vi "Test_User_Event.vi"() -> ()   [LabVIEW 2014, in "User_Event_Library.lvlib"]
uses:
  User_Event_Library.lvlib
  Send_User_Event_Array.vi
panel:
  out "number (0 to 1)":dbl(graph)
  in  "Blank Button":bool
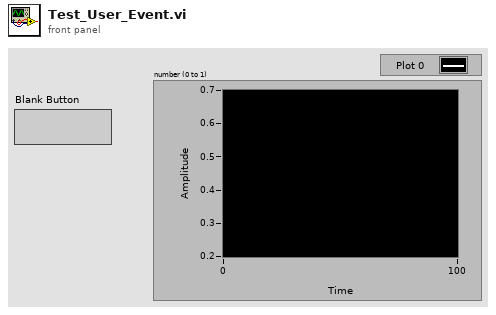
[diagram p1: front panel]
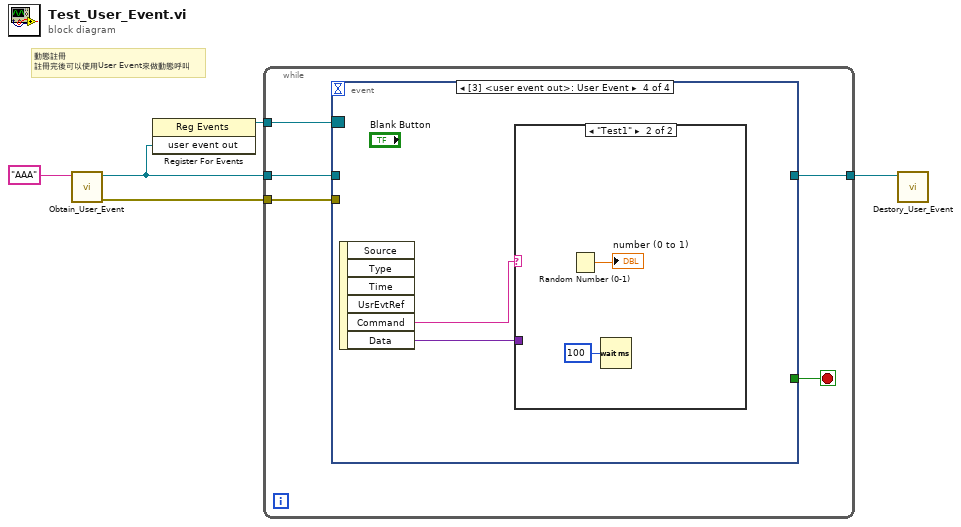
[diagram p0: block diagram]
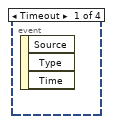
[diagram p2: hidden frame]
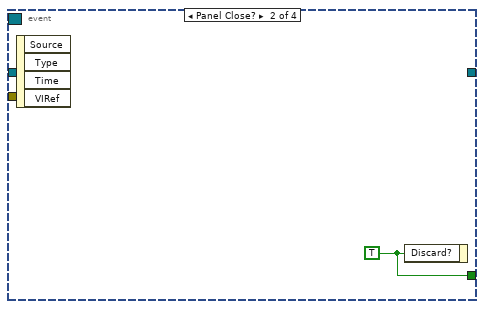
[diagram p3: hidden frame]
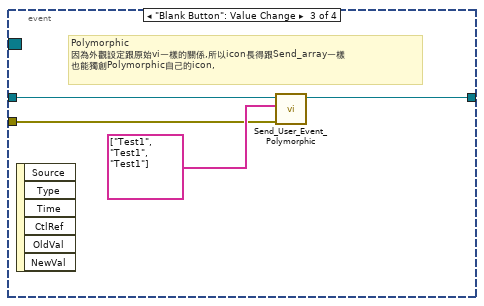
[diagram p4: hidden frame]
diagram:
  # "動態註冊\n註冊完後可以使用User Event來做動態呼叫"
  n1 = call "Obtain_User_Event.vi"("Name"="AAA" ("Command")) -> ("error out"=w4:errorcluster, "user event out"=w2:refnum<user-event>)  [unwired: 9 in]
  n2 = register-events(w2) -> (reference out=w1:refnum<event-registration>)  [unwired: 2 in, 1 out]
  n3 = while {
    tunnel: w2 -> [w8]
    tunnel: [w9] -> w5
    tunnel: w4 -> [w7]
    tunnel: w1 -> [w6]
    stop <- w10 stop-if-true
    n4 = event shown="[3] <user event out>: User Event" {
      selector: w6 -> [_ _ _ _]
      dyn-events: _ -> [_ _ _ _]
      timeout: _ -> [_ _ _ _]
      tunnel: [_ w11 _ _] -> w10
      tunnel: [_ _ w12 _] -> w9
      tunnel: w8 -> [_ _ w15 _]
      tunnel: w7 -> [_ _ w13 _]
      event Timeout {
        n5 = event-data() -> ()  [unwired: 1 in, 3 out]
      }
      event Panel Close? {
        w11 = TRUE ("Discard?")
        n6 = event-data() -> ()  [unwired: 1 in, 4 out]
        n7 = event-data("Discard?"=w11) -> ()  [unwired: 1 in, 1 out]
      }
      event "Blank Button": Value Change {
        # "Polymorphic\n因為外觀設定跟原始vi一樣的關係,所以icon長得跟Send_array一樣\n也能獨創Polymorphic自己的icon,"
        n8 = event-data() -> ()  [unwired: 1 in, 6 out]
        n9 = call-poly "Send_User_Event_Polymorphic.vi"("error in (no error)"=w13, "Command"=string[] ["Test1", "Test1", "Test1"], "user event In"=w15) -> ("user event Out"=w12:refnum<user-event>)  [unwired: 7 in, 1 out]
      }
      event User Event {
        n10 = event-data() -> ("Command"=w17:string, "Data"=w16:variant)  [unwired: 1 in, 4 out]
        n11 = case shown="\"Test1\"" w17 {
          tunnel: w16 -> [_ _]
          frame "False", Default {
          }
          frame "Test1" {
            n12 = Random Number (0-1)() -> (number: 0 to 1=→"number (0 to 1)":dbl)
            n13 = Wait (ms)(milliseconds to wait=u32 100) -> ()  [unwired: 1 out]
          }
        }
      }
    }
  }
  n14 = call "Destory_User_Event.vi"("user event In"=w5) -> ()  [unwired: 10 in, 1 out]
